vi "Set Col-Row ROI.vi"(9 "ROI Rows":cluster{"Index":u32, "Length":u32}, 10 "ROI Cols":cluster{"Index":u32, "Length":u32}, 11 "Base Graph in":refnum<class "Base Graph.lvclass">) -> (3 "Base Graph out":refnum<class "Base Graph.lvclass">)   [LabVIEW 2023, in "Base Graph.lvclass"]
uses:
  Base Graph.lvclass
  Base Graph.lvclass/Base Graph.ctl
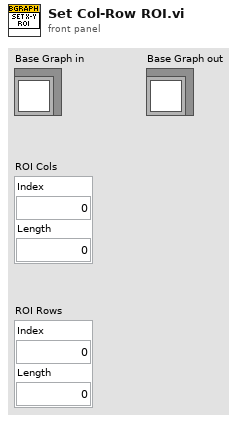
[diagram p1: front panel]
types:
  T1 = cluster{"ROI Cols":cluster{"Index":u32, "Length":u32}, "ROI Rows":cluster{"Index":u32, "Length":u32}}
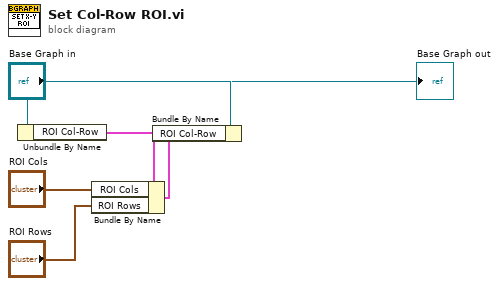
[diagram p0: block diagram]
diagram:
  n1 = Unbundle By Name("Base Graph in") -> ("ROI Col-Row"=w2:T1)
  n2 = Bundle By Name(cluster=w2, "ROI Cols"="ROI Cols", "ROI Rows"="ROI Rows") -> (w1:T1)
  n3 = Bundle By Name(cluster="Base Graph in", "ROI Col-Row"=w1) -> (→"Base Graph out":refnum<class "Base Graph.lvclass">)
